vi "Default Config Data.vi"() -> (5 "Default Data":T1)   [LabVIEW 2015, in "App Config.lvlib"]
uses:
  App Config.lvlib
  App Config Data.ctl
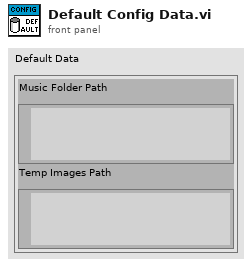
[diagram p1: front panel]
types:
  T1 = typedef "App Config.lvlib/App Config Data.ctl" = cluster{"Music Folder Path":path, "Temp Images Path":path}
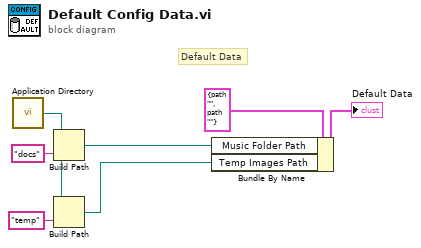
[diagram p0: block diagram]
diagram:
  # "Default Data"
  n1 = call <vilib>:"Application Directory.vi"() -> ("Application Directory"=w2:path)
  n2 = Build Path(base path=w2, name or relative path="docs") -> (appended path=w5:path)
  n3 = Build Path(base path=w2, name or relative path="temp") -> (appended path=w1:path)
  n4 = Bundle By Name(cluster=T1 {"Music Folder Path"=path "", "Temp Images Path"=path ""} ("Data"), "Music Folder Path"=w5, "Temp Images Path"=w1) -> (→"Default Data":T1)
